vi "SLSC Session Daemon.vi"(8 "error in (no error)":errorcluster, 11 "device":refnum<k21>) -> (0 "error out":errorcluster)   [LabVIEW 2015, in "SLSC Switch.lvlib" / "SLSC Session.lvclass"]
uses:
  SLSC Session/SLSC Session.lvclass
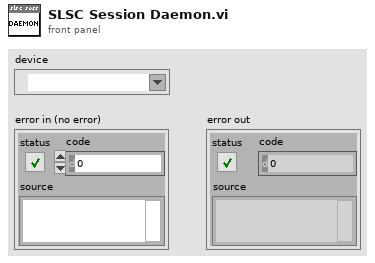
[diagram p1: front panel]
types:
  T1 = typedef "SLSC Switch.lvlib/SLSC Session.lvclass/Session Handle.ctl" = refnum<data-value>
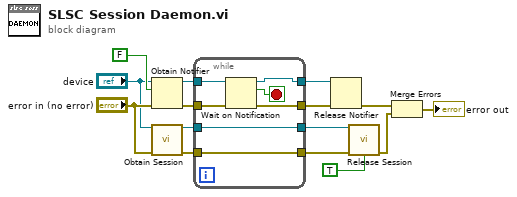
[diagram p0: block diagram]
diagram:
  n1 = Obtain Notifier(name (unnamed)="device", notification data type=FALSE, error in (no error)="error in (no error)") -> (notifier out=w14:refnum<notifier>, error out=w9:errorcluster)  [unwired: 1 in, 1 out]
  n2 = call "Obtain Session.vi"("device"="device", "error in (no error)"="error in (no error)") -> ("Session Handle"=w15:T1, "error out"=w11:errorcluster)  [unwired: 12 in]
  n3 = while {
    tunnel: w15 -> [w20]
    tunnel: w14 -> [w22]
    tunnel: [w20] -> w12
    tunnel: w11 -> [w19]
    tunnel: [w19] -> w10
    tunnel: w9 -> [w18]
    tunnel: [w17] -> w4
    tunnel: [w16] -> w2
    stop <- w21 stop-if-true
    n4 = Wait on Notification(notifier=w22, error in (no error)=w18) -> (notifier out=w16:refnum<notifier>, notification=w21:bool, error out=w17:errorcluster)  [unwired: 2 in, 1 out]
  }
  n5 = Release Notifier(notifier=w2, error in (no error)=w4) -> (error out=w3:errorcluster)  [unwired: 1 in, 2 out]
  n6 = call "Release Session.vi"("Session Handle"=w12, "error in (no error)"=w10, "force destroy? (F)"=TRUE) -> ("error out"=w8:errorcluster)  [unwired: 12 in]
  n7 = Merge Errors(w3, w8) -> (→"error out":errorcluster)
